vi "sales data (SubVI).vi"() -> (3 "sales data":string[][](array[string]))   [LabVIEW 2020]
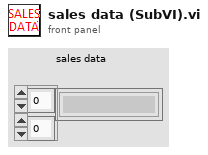
[diagram p1: front panel]
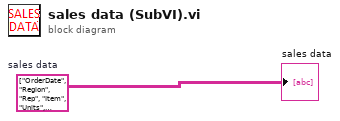
[diagram p0: block diagram]
diagram:
  w1 = string[][] [["OrderDate", "Region", "Rep", "Item", "Units", "UnitCost"], ["1/6/2016", "East", "Jones", "Pencil", "95", "1.99"], ["1/23/2016", "Central", "Kivell", "Binder", "50", "19.99"], ["2/9/2016", "Central", "Jardine", "Pencil", "36", "4.99"], ["2/26/2016", "Central", "Gill", "Pen", "27", "19.99"], ["3/15/2016", "West", "Sorvino", "Pencil", "56", "2.99"], ["4/1/2016", "East", "Jones", "Binder", "60", "4.99"], ["4/18/2016", "Central", "Andrews", "Pencil", "75", "1.99"], ["5/5/2016", "Central", "Jardine", "Pencil", "90", "4.99"], ["5/22/2016", "West", "Thompson", "Pencil", "32", "1.99"], ["6/8/2016", "East", "Jones", "Binder", "60", "8.99"], ["6/25/2016", "Central", "Morgan", "Pencil", "90", "4.99"], ["7/12/2016", "East", "Howard", "Binder", "29", "1.99"], ["7/29/2016", "East", "Parent", "Binder", "81", "19.99"], ["8/15/2016", "East", "Jones", "Pencil", "35", "4.99"], ["9/1/2016", "Central", "Smith", "Desk", "2", "125"], ["9/18/2016", "East", "Jones", "Pen Set", "16", "15.99"], ["10/5/2016", "Central", "Morgan", "Binder", "28", "8.99"], ["10/22/2016", "East", "Jones", "Pen", "64", "8.99"], ["11/8/2016", "East", "Parent", "Pen", "15", "19.99"], ["11/25/2016", "Central", "Kivell", "Pen Set", "96", "4.99"], ["12/12/2016", "Central", "Smith", "Pencil", "67", "1.29"], ["12/29/2016", "East", "Parent", "Pen Set", "74", "15.99"], ["1/15/2017", "Central", "Gill", "Binder", "46", "8.99"], ["2/1/2017", "Central", "Smith", "Binder", "87", "15"], ["2/18/2017", "East", "Jones", "Binder", "4", "4.99"], ["3/7/2017", "West", "Sorvino", "Binder", "7", "19.99"], ["3/24/2017", "Central", "Jardine", "Pen Set", "50", "4.99"], ["4/10/2017", "Central", "Andrews", "Pencil", "66", "1.99"], ["4/27/2017", "East", "Howard", "Pen", "96", "4.99"], ["5/14/2017", "Central", "Gill", "Pencil", "53", "1.29"], ["5/31/2017", "Central", "Gill", "Binder", "80", "8.99"], ["6/17/2017", "Central", "Kivell", "Desk", "5", "125"], ["7/4/2017", "East", "Jones", "Pen Set", "62", "4.99"], ["7/21/2017", "Central", "Morgan", "Pen Set", "55", "12.49"], ["8/7/2017", "Central", "Kivell", "Pen Set", "42", "23.95"], ["8/24/2017", "West", "Sorvino", "Desk", "3", "275"], ["9/10/2017", "Central", "Gill", "Pencil", "7", "1.29"], ["9/27/2017", "West", "Sorvino", "Pen", "76", "1.99"], ["10/14/2017", "West", "Thompson", "Binder", "57", "19.99"], ["10/31/2017", "Central", "Andrews", "Pencil", "14", "1.29"], ["11/17/2017", "Central", "Jardine", "Binder", "11", "4.99"], ["12/4/2017", "Central", "Jardine", "Binder", "94", "19.99"], ["12/21/2017", "Central", "Andrews", "Binder", "28", "4.99"]]  # sales data
  "sales data" <- w1
